vi "Send Set Output Lines.vi"(7 "Message Priority (Normal)":T1=enum."Normal", 8 "error in (no error)":errorcluster, 9 "Start Index":i32, 10 "DO Lines":bool[](array[boolean]), 11 "Message Enqueuer":refnum<class "Message Enqueuer.lvclass">) -> (0 "error out":errorcluster, 3 "Message Enqueuer out":refnum<class "Message Enqueuer.lvclass">)   [LabVIEW 2020, in "BNT_ULx.lvlib" / "Set Output Lines Msg.lvclass"]
doc: "Sends the <B>BNT_ULx.lvlib:Set Output Lines Msg.lvclass</B> message.\n\n<B>BNT_DAQmx.lvlib:BNT_DAQmx-MCSV.lvclass:Set Output Lines.vi</B> Description:\n\nWrite line values to DAQmx device and publish.\n\nTimeout is set to constant 1s."
uses:
  Set Output Lines Msg.lvclass
  <vilib>/ActorFramework/Message Enqueuer/Message Enqueuer.lvclass
  C:/Program Files (x86)/National Instruments/LabVIEW 2020/vi.lib/ActorFramework/Message/Message.lvclass
  <vilib>/ActorFramework/Message Enqueuer/Message Priority.ctl
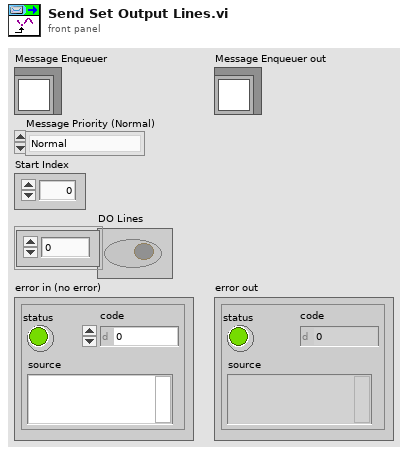
[diagram p1: front panel]
types:
  T1 = typedef "Actor Framework.lvlib/Message Enqueuer.lvclass/Message Priority.ctl" = enum16{"Low", "Normal", "High"}
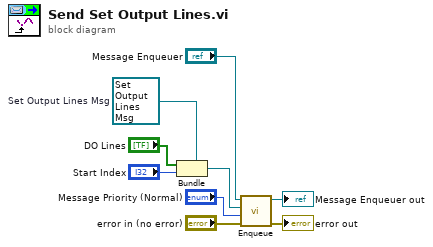
[diagram p0: block diagram]
diagram:
  w3 = refnum<class "Set Output Lines Msg.lvclass"> refnum  # Set Output Lines Msg
  n1 = Bundle(cluster=w3, "DO Lines", "Start Index") -> (w6:refnum<class "Set Output Lines Msg.lvclass">)
  n2 = call <vilib>:"Enqueue.vi"("error in (no error)"="error in (no error)", "Message Priority (Normal)"="Message Priority (Normal)", "Message"=w6, "Message Enqueuer in"="Message Enqueuer") -> ("error out"=→"error out":errorcluster, "Message Enqueuer out"=→"Message Enqueuer out":refnum<class "Message Enqueuer.lvclass">)  [unwired: 6 in]
